vi "EventLog.FormatErrorMessage.vi"(1 "Error string in":string) -> (0 "Error string out":string)   [LabVIEW 2016]
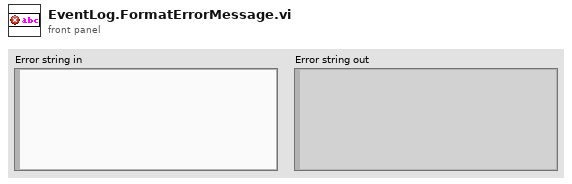
[diagram p1: front panel]
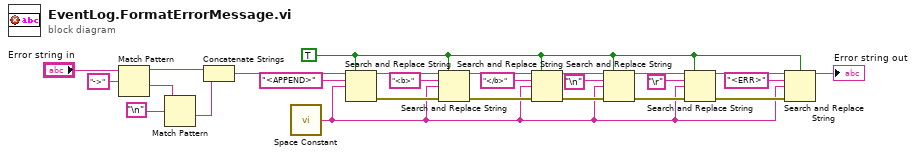
[diagram p0: block diagram]
diagram:
  w4 = TRUE ("replace all? (F)")
  n1 = Match Pattern(string="Error string in", regular expression="->") -> (before substring=w22:string, after substring=w24:string)  [unwired: 1 in, 2 out]
  n2 = Match Pattern(string=w24, regular expression="\n") -> (after substring=w21:string)  [unwired: 1 in, 3 out]
  n3 = Concatenate Strings(w22, w21) -> (w8:string)
  n4 = call <vilib>:"Space Constant.vi"() -> ("String"=w2:string)
  n5 = Search and Replace String(replace all?=w4, input string=w8, search string="<APPEND>", replace string=w2) -> (result string=w19:string, error out=w13:errorcluster)  [unwired: 4 in, 2 out]
  n6 = Search and Replace String(replace all?=w4, input string=w19, search string="<b>", replace string=w2, error in=w13) -> (result string=w18:string, error out=w14:errorcluster)  [unwired: 3 in, 2 out]
  n7 = Search and Replace String(replace all?=w4, input string=w18, search string="</b>", replace string=w2, error in=w14) -> (result string=w15:string, error out=w16:errorcluster)  [unwired: 3 in, 2 out]
  n8 = Search and Replace String(replace all?=w4, input string=w15, search string="\n", replace string=w2, error in=w16) -> (result string=w10:string, error out=w9:errorcluster)  [unwired: 3 in, 2 out]
  n9 = Search and Replace String(replace all?=w4, input string=w10, search string="\r", replace string=w2, error in=w9) -> (result string=w6:string, error out=w3:errorcluster)  [unwired: 3 in, 2 out]
  n10 = Search and Replace String(case sensitive?=w4, input string=w6, search string="<ERR>", replace string=w2, error in=w3) -> (result string=→"Error string out":string)  [unwired: 3 in, 3 out]
